vi "F帧解析.vi"(3 "10输入":string[](array[string]), 5 "F输入数组":dbl[](array[numeric])) -> (0 "10":string[](array[string]), 1 "F":string[](array[string]))   [LabVIEW 2013]
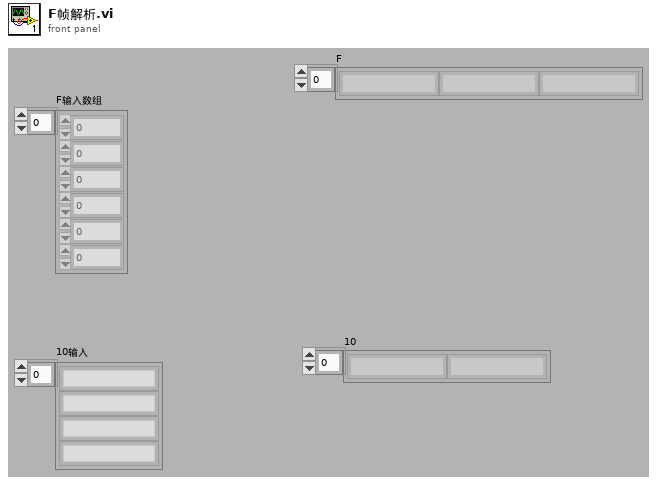
[diagram p1: front panel]
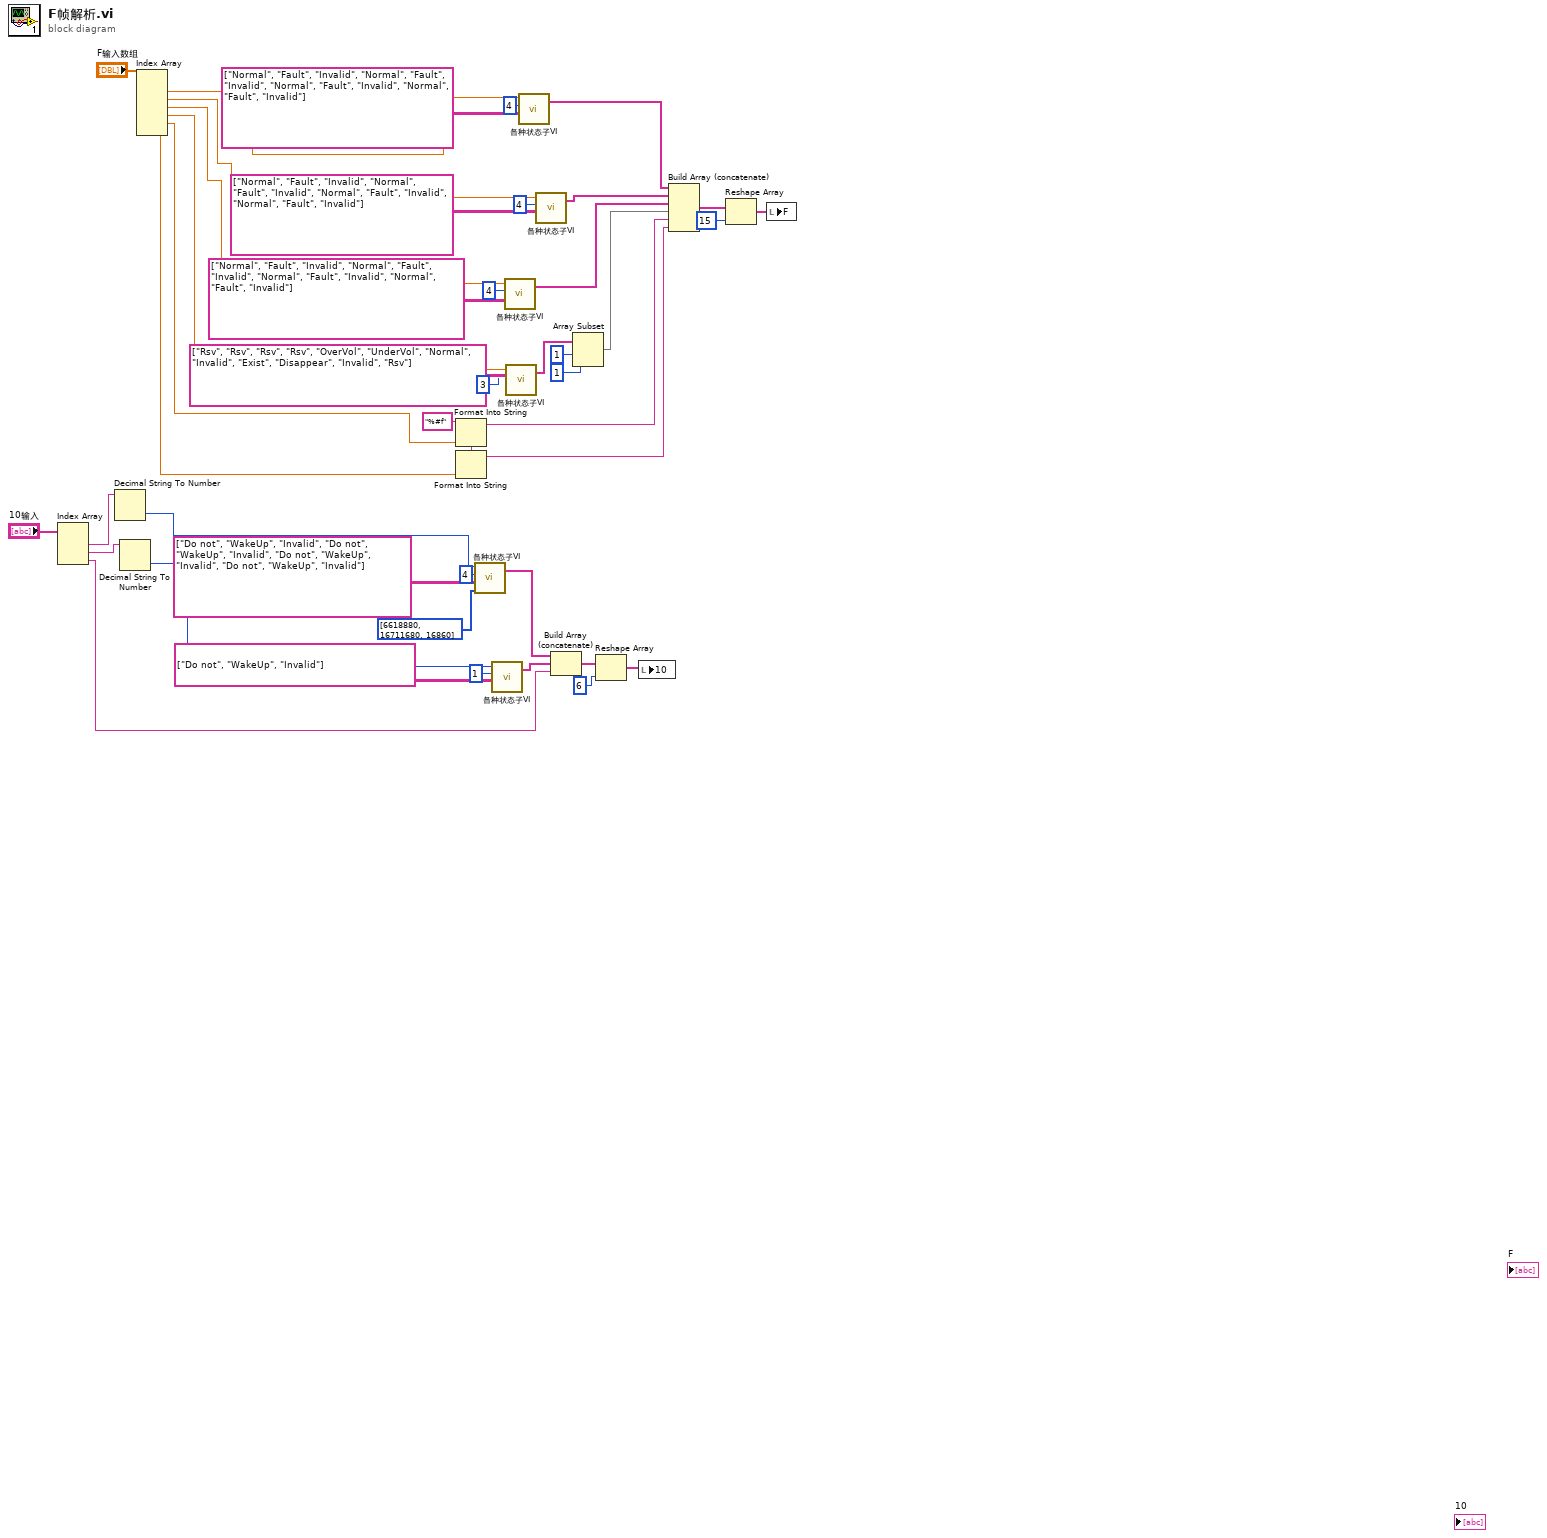
[diagram p0: block diagram]
diagram:
  w36 = "%#f" ("格式字符串")
  n1 = Index Array(array="10输入") -> (element #1=w13:string, element #2=w12:string, element #3=w11:string)  [unwired: 3 in]
  n2 = Decimal String To Number(string=w13) -> (number=w10:i32)  [unwired: 3 out]
  n3 = Decimal String To Number(string=w12) -> (number=w9:i32)  [unwired: 3 out]
  n4 = Index Array(array="F输入数组") -> (element #1=w8:dbl, element #2=w7:dbl, element #3=w6:dbl, element #4=w5:dbl, element #5=w2:dbl, element #6=w1:dbl)  [unwired: 6 in]
  n5 = Format Into String(format string=w36, w2) -> (resulting string=w37:string)  [unwired: 2 in, 1 out]
  n6 = Format Into String(format string=w36, w1) -> (resulting string=w38:string)  [unwired: 2 in, 1 out]
  n7 = call "各种状态子VI.vi"("颜色输入"=u32[] [6618880, 16711680, 16860], "状态输入"=string[][] [["Do not", "WakeUp", "Invalid"], ["Do not", "WakeUp", "Invalid"], ["Do not", "WakeUp", "Invalid"], ["Do not", "WakeUp", "Invalid"]], "几种类型"=4, "数值"=w10) -> ("状态"=w19:string[])  [unwired: 1 out]
  n8 = call "各种状态子VI.vi"("状态输入"=string[][] [["Do not", "WakeUp", "Invalid"]], "几种类型"=1, "数值"=w9) -> ("状态"=w20:string[])  [unwired: 1 in, 1 out]
  n9 = call "各种状态子VI.vi"("状态输入"=string[][] [["Normal", "Fault", "Invalid"], ["Normal", "Fault", "Invalid"], ["Normal", "Fault", "Invalid"], ["Normal", "Fault", "Invalid"]], "几种类型"=4, "数值"=w6) -> ("状态"=w31:string[])  [unwired: 1 in, 1 out]
  n10 = call "各种状态子VI.vi"("状态输入"=string[][] [["Rsv", "Rsv", "Rsv", "Rsv"], ["OverVol", "UnderVol", "Normal", "Invalid"], ["Exist", "Disappear", "Invalid", "Rsv"]], "几种类型"=3, "数值"=w5) -> ("状态"=w39:string[])  [unwired: 1 in, 1 out]
  n11 = call "各种状态子VI.vi"("状态输入"=string[][] [["Normal", "Fault", "Invalid"], ["Normal", "Fault", "Invalid"], ["Normal", "Fault", "Invalid"], ["Normal", "Fault", "Invalid"]], "几种类型"=4, "数值"=w8) -> ("状态"=w29:string[])  [unwired: 1 in, 1 out]
  n12 = call "各种状态子VI.vi"("状态输入"=string[][] [["Normal", "Fault", "Invalid"], ["Normal", "Fault", "Invalid"], ["Normal", "Fault", "Invalid"], ["Normal", "Fault", "Invalid"]], "几种类型"=4, "数值"=w7) -> ("状态"=w30:string[])  [unwired: 1 in, 1 out]
  n13 = Build Array (concatenate)(w19, w20, w11) -> (w22:string[])
  n14 = Array Subset(array=w39, index=1 ("索引"), length=1 ("长度")) -> (w42:string[])
  n15 = Reshape Array(w22, 6 ("维数大小")) -> (w3:string[])
  n16 = local write "10"(w3) -> ()
  n17 = Build Array (concatenate)(w29, w30, w31, w42, w37, w38) -> (w43:string[])
  n18 = Reshape Array(w43, 15 ("维数大小")) -> (w4:string[])
  n19 = local write "F"(w4) -> ()
